vi "Update Plugin Test End Result.vi"(10 "Result":T1, 11 "Execution UI in":refnum<class "Execution UI.lvclass">) -> (3 "Execution UI out":refnum<class "Execution UI.lvclass">)   [LabVIEW 2020, in "Execution UI.lvclass"]
uses:
  Execution UI.lvclass
  Core/Result/Result.ctl
  Core/Result/Status.ctl
  Core/Result/Type.ctl
  Execution UI.lvclass/Execution UI.ctl
  Framework/Plugin/Plugin.lvclass
  Core/Result/Result.lvlib
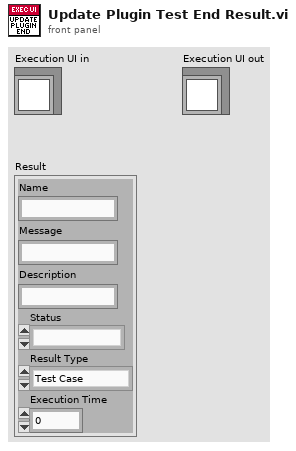
[diagram p1: front panel]
types:
  T1 = typedef "Result.lvlib/Result.ctl" = cluster{"Name":string, "Message":string, "Description":string, "Status":T2, "Result Type":T3, "Execution Time":dbl}
  T2 = typedef "Result.lvlib/Status.ctl" = enum16{"", "Passed", "Failed", "Error", "Skipped", "Setup Error", "Broken", "Teardown Error"}
  T3 = typedef "Result.lvlib/Type.ctl" = enum16{"Test Case", "Test Suite", "Test Run", "Pass", "Fail", "Skip", "Pass if", "Fail if", "Pass if Error", "Fail if Error", "Pass if Equal", "Fail if Equal"}
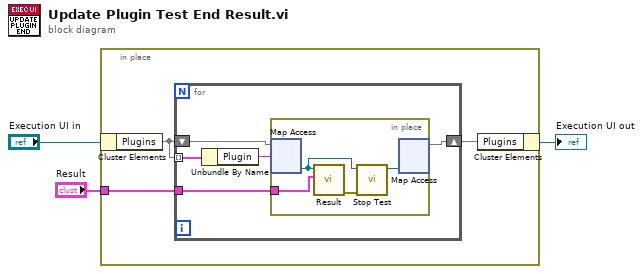
[diagram p0: block diagram]
diagram:
  n1 = in-place {
    in-place-border: "Result" -> [w6]
    n2 = in-place-cluster #1("Execution UI in") -> ("Plugins"=w4:map{string, refnum<class "Plugin.lvclass">})
    n3 = for {
      tunnel: w6 -> [w8]
      shift-right: [w7] -> w5
      shift-left: w4 -> [w11]
      tunnel: w4 -> [w10] mode=indexing
      n4 = Unbundle By Name(w10) -> ("Plugin"=w9:string)
      n5 = in-place {
        in-place-border: w8 -> [w15]
        n6 = in-place-map #2(w11, w9) -> (w13:refnum<class "Plugin.lvclass">)  [unwired: 1 in, 1 out]
        n7 = call-dynamic "Result.vi"("Result"=w15, "Plugin In"=w13) -> ("error out"=w14:errorcluster)  [unwired: 9 in]
        n8 = call-dynamic "Stop Test.vi"("error in (no error)"=w14, "Plugin in"=w13) -> ("Plugin out"=w12:refnum<class "Plugin.lvclass">)  [unwired: 8 in, 1 out]
        n9 = in-place-map #2(w12) -> (w7:map{string, refnum<class "Plugin.lvclass">})  [unwired: 1 in, 2 out]
      }
    }
    n10 = in-place-cluster #1("Plugins"=w5) -> (→"Execution UI out":refnum<class "Execution UI.lvclass">)
  }
